vi "Timer Is Time Up.vi"(5 "Finish Time":timestamp) -> (0 "Time left (ms)":dbl, 1 "Time left (S)":dbl, 2 "Time Complete":bool)   [LabVIEW 2020]
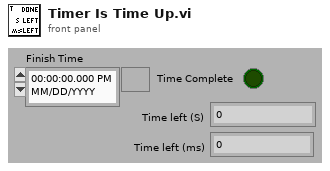
[diagram p1: front panel]
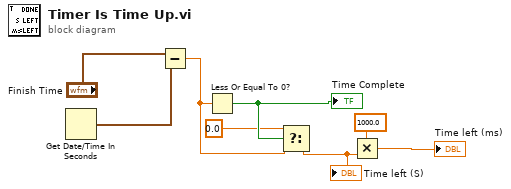
[diagram p0: block diagram]
diagram:
  n1 = Get Date/Time In Seconds() -> (seconds since 1Jan1904=w5:timestamp)
  n2 = Subtract(x="Finish Time", y=w5) -> (x-y=w2:dbl)
  n3 = Less Or Equal To 0?(x=w2) -> (x <= 0?=w4:bool)
  "Time Complete" <- w4
  n4 = Select(t=0.0, s=w4, f=w2) -> (s? t:f=w1:dbl)
  "Time left (S)" <- w1
  n5 = Multiply(x=1000.0, y=w1) -> (x*y=→"Time left (ms)":dbl)
